vi "Write State.vi"(8 "error in (no error)":errorcluster, 10 "State":string, 11 "TCS in":refnum<class "TCS.lvclass">) -> (0 "error out":errorcluster, 3 "TCS out":refnum<class "TCS.lvclass">)   [LabVIEW 2018, in "TCS.lvclass"]
uses:
  TCS.lvclass
  TCS.lvclass/TCS.ctl
  State Machine/State Machine.lvclass
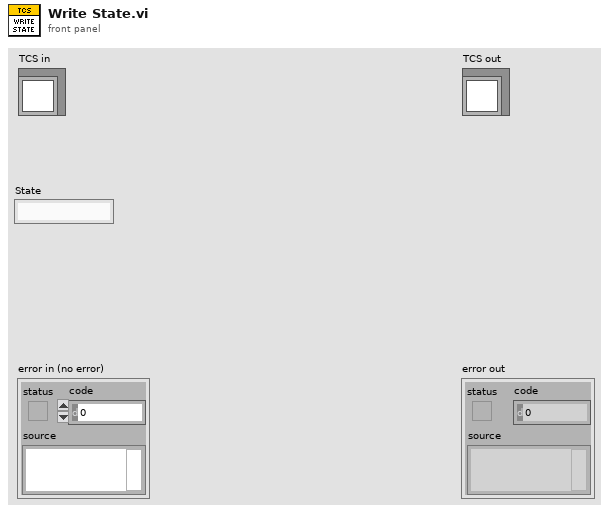
[diagram p1: front panel]
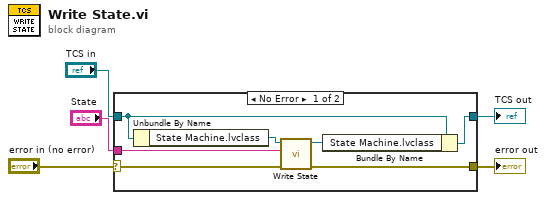
[diagram p0: block diagram]
diagram:
  n1 = case shown="No Error" "error in (no error)" {
    selector: "error in (no error)" -> [w8 w14]
    tunnel: [w7 w14] -> w4
    tunnel: [w10 w13] -> w2
    tunnel: "TCS in" -> [w11 w13]
    tunnel: "State" -> [w6 _]
    frame No Error {
      n2 = Unbundle By Name(w11) -> ("State Machine.lvclass"=w12:refnum<class "State Machine.lvclass">)
      n3 = call-dynamic "Write State.vi"("error in (no error)"=w8, "State"=w6, "State Machine in"=w12) -> ("error out"=w7:errorcluster, "State Machine out"=w9:refnum<class "State Machine.lvclass">)  [unwired: 7 in]
      n4 = Bundle By Name(cluster=w11, "State Machine.lvclass"=w9) -> (w10:refnum<class "TCS.lvclass">)
    }
    frame Error {
    }
  }
  "error out" <- w4
  "TCS out" <- w2
